vi "Stop and Close FPGA.vi"(8 "error in (no error)":errorcluster, 11 "FPGA VI Reference In":T1) -> (0 "error out":errorcluster)   [LabVIEW 2018, in "RT-FPGA Interface API.lvlib"]
uses:
  RT-FPGA Interface API.lvlib
  <vilib>/rvi/interface/nirviReadWriteControl/nirviReadWriteControl.xnode
  <vilib>/rvi/interface/nirviCloseFPGA/nirviCloseFPGA.xnode
  FPGA ref.ctl
  NiFpgaLv.dll
  <vilib>/Utility/error.llb/Error Cluster From Error Code.vi
  <vilib>/rvi/interface/Simulation/niFpgaSimulationCallBeginRW.vi
  <vilib>/rvi/errors/niLvFpgaAdjustHostInterfaceError.vi
  <vilib>/FPGAPlugInAG/Dynamic/niLvFpga_Close_Dynamic.vi
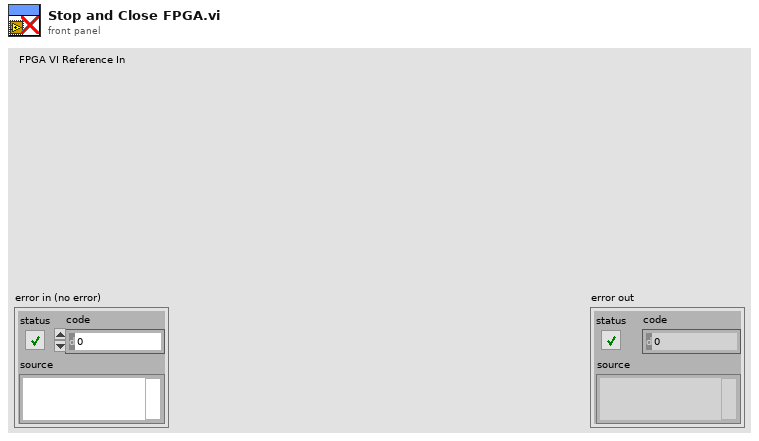
[diagram p1: front panel]
types:
  T1 = typedef "RT-FPGA Interface API.lvlib/FPGA ref.ctl" = refnum<k20>
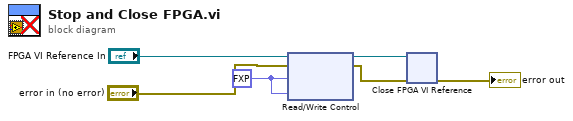
[diagram p0: block diagram]
diagram:
  w6 = fxp<+/-,20,5> 0.0 ("Bomba 1")
  n1 = xnode "Read/Write Control"("FPGA VI Reference In"="FPGA VI Reference In", "error in"="error in (no error)", "Bomba 1"=w6, "Bomba 2"=w6) -> ("FPGA VI Reference Out"=w5:T1, "error out"=w4:errorcluster)
  n2 = xnode "Close FPGA VI Reference"("FPGA VI Reference In"=w5, "error in"=w4) -> ("error out"=→"error out":errorcluster)
